vi "BTK conductivity.vi"(8 "error in":errorcluster, 9 "dx":dbl=1.0 format="%0.2f", 10 "Current":dbl[](array[numeric])) -> (0 "error out":errorcluster, 2 "Conductivity":dbl[](array[numeric]))   [LabVIEW 2021]
uses:
  <vilib>/Analysis/NI_AALPro.lvlib
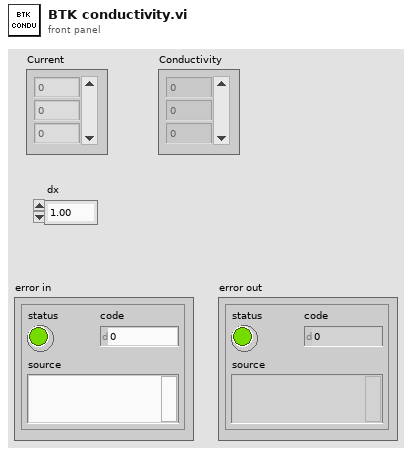
[diagram p1: front panel]
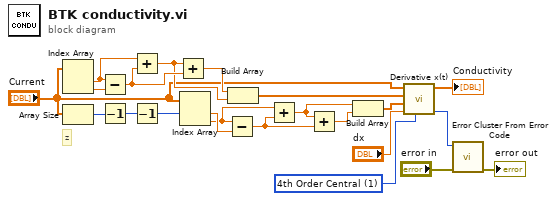
[diagram p0: block diagram]
diagram:
  w5 = u16 1 items=["2nd Order Central", "4th Order Central", "Forward", "Backward"] ("method")
  # "z"
  n1 = Index Array(array="Current") -> (element #1=w20:dbl, element #2=w21:dbl)  [unwired: 2 in]
  n2 = Array Size(array="Current") -> (size(s)=w22:i32)
  n3 = Subtract(x=w20, y=w21) -> (x-y=w19:dbl)
  n4 = Decrement(x=w22) -> (x-1=w17:i32)
  n5 = Add(x=w20, y=w19) -> (x+y=w9:dbl)
  n6 = Decrement(x=w17) -> (x-1=w16:i32)
  n7 = Add(x=w9, y=w19) -> (x+y=w8:dbl)
  n8 = Index Array(array="Current", index #1=w16) -> (element #1=w12:dbl, element #2=w11:dbl)  [unwired: 1 in]
  n9 = Subtract(x=w11, y=w12) -> (x-y=w13:dbl)
  n10 = Build Array(w8, w9) -> (w18:dbl[])
  n11 = Add(x=w11, y=w13) -> (x+y=w14:dbl)
  n12 = Add(x=w14, y=w13) -> (x+y=w15:dbl)
  n13 = Build Array(w14, w15) -> (w10:dbl[])
  n14 = call <vilib>:"Derivative x(t).vi"("method"=w5, "dt"="dx", "Final Condition"=w10, "Initial Condition"=w18, "X"="Current") -> ("error"=w3:i32, "dX/dt"=→"Conductivity":dbl[])  [unwired: 5 in]
  n15 = call <vilib>:"Error Cluster From Error Code.vi"("error in (no error)"="error in", "error code (0)"=w3) -> ("error out"=→"error out":errorcluster)  [unwired: 7 in]
